vi "Server FGV.vi"(7 "Mode (Get All)":T2=enum."Get All", 8 "error in (no error)":errorcluster, 11 "Stock Name":string) -> (0 "error out":errorcluster, 2 "purchase price":dbl, 3 "Full Features MCP Server Data":T1)   [LabVIEW 2025, in "Full Featured MCP Server.lvlib"]
doc: "This FGV contains the data for the stock market server. It makes sure no race-conditions happen when accessing the data in the main.vi and the mcp tools simultaneously."
uses:
  Server FGV Modes.ctl
  Server Data.ctl
  <vilib>/Utility/error.llb/Error Cluster From Error Code.vi
  <vilib>/ErrorRing/Error Ring.xnode
  Full Featured MCP Server.lvlib
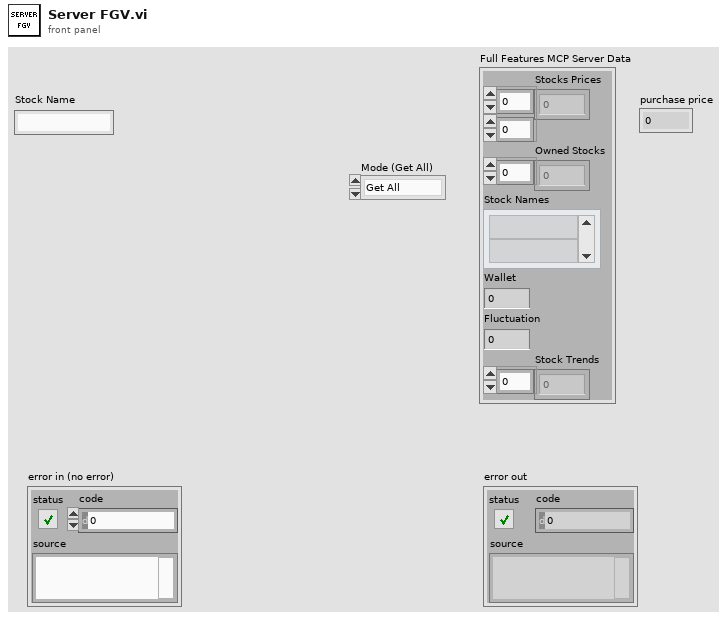
[diagram p1: front panel]
types:
  T1 = typedef "Full Featured MCP Server.lvlib/Server Data.ctl" = cluster{"Stocks Prices":dbl[][], "Owned Stocks":i32[], "Stock Names":string[], "Wallet":dbl, "Fluctuation":dbl, "Stock Trends":dbl[]}
  T2 = typedef "Full Featured MCP Server.lvlib/Server FGV Modes.ctl" = enum16{"Update Stocks", "Buy Stock", "Get All", "Init"}
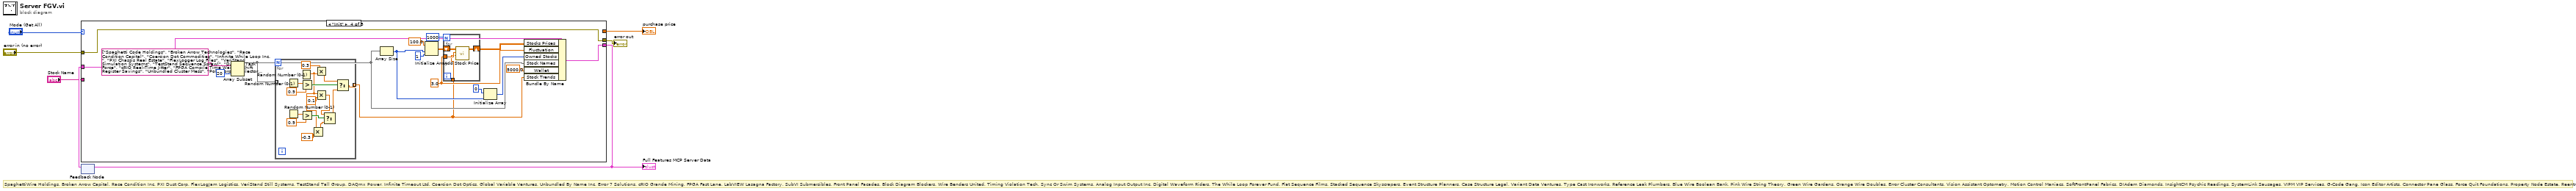
[diagram p0: block diagram]
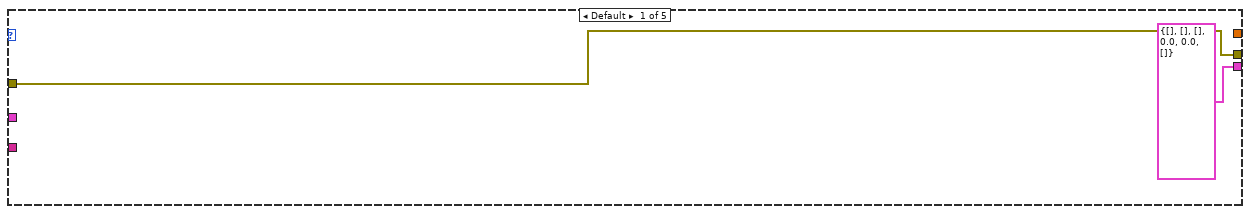
[diagram p2: hidden frame]
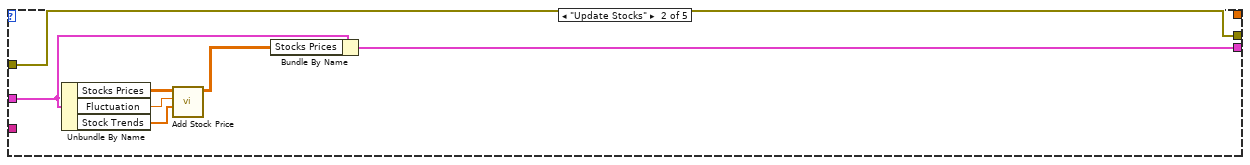
[diagram p3: hidden frame]
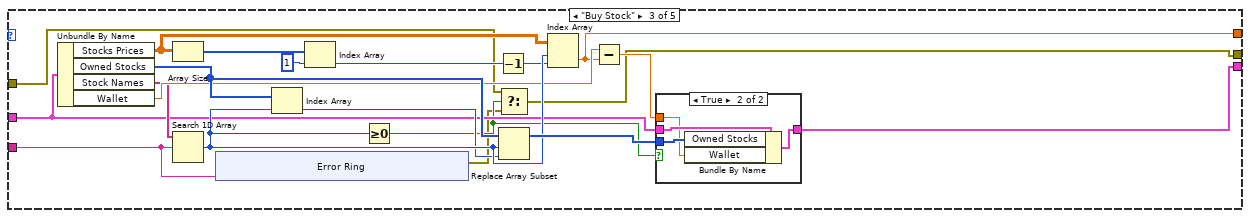
[diagram p4: hidden frame]
diagram:
  # "SpaghettiWire Holdings, Broken Arrow Capital, Race Condition Inc, PXI Dust Corp, FlexLogJam Logistics, VeriStand Still Systems, TestStand Tall Group, DAQmx Power, Infinite Timeout Ltd, Coercion Dot Optics, Global Variable Ventures, Unbundled By Name Inc, Error 7 Solutions, cRIO Grande Mining, FPGA Fast Lane, LabVIEW Lasagna Factory, SubVI Submersibles, Front Panel Facades, Block Diagram Blockers, Wire Benders United, Timing Violation Tech, Sync Or Swim Systems, Analog Input Output Inc, Digital Waveform Riders, The While Loop Forever Fund, Flat Sequence Films, Stacked Sequence Skyscrapers, Event Structure Planners, Case Structure Legal, Variant Data Ventures, Type Cast Ironworks, Reference Leak Plumbers, Blue Wire Boolean Bank, Pink Wire String Theory, Green Wire Gardens, Orange Wire Doubles, Error Cluster Consultants, Vision Assistant Optometry, Motion Control Maniacs, SoftFrontPanel Fabrics, DIAdem Diamonds, InsightCM Psychic Readings, SystemLink Sausages, VIPM VIP Services, G-Code Gang, Icon Editor Artists, Connector Pane Glass, Force Quit Foundations, Property Node Estate, Reentrant Execution Groups"
  n1 = feedback #1() -> (w6:T1)  [unwired: 1 in]
  n2 = case shown="\"Init\"" "Mode (Get All)" {
    tunnel: [T1 {"Stocks Prices"=[], "Owned Stocks"=[], "Stock Names"=[], "Wallet"=0.0, "Fluctuation"=0.0, "Stock Trends"=[]} ("Full Features MCP Server Data") w16 w24 w63 w86] -> w5
    tunnel: w6 -> [_ w15 w23 w65 w86]
    tunnel: "Stock Name" -> [_ _ w17 _ _]
    tunnel: [_ _ w22 _ _] -> w3
    tunnel: "error in (no error)" -> [w8 w11 w21 w64 w85]
    tunnel: [w8 w11 w20 w64 w85] -> w1
    frame Default {
    }
    frame "Update Stocks" {
      n3 = Unbundle By Name(w15) -> ("Stocks Prices"=w14:dbl[][], "Fluctuation"=w13:dbl, "Stock Trends"=w10:dbl[])
      n4 = call "Add Stock Price.vi"("Trends"=w10, "Fluctuation"=w13, "Stocks Prices"=w14) -> ("Stock Prices out"=w12:dbl[][])  [unwired: 8 in]
      n5 = Bundle By Name(cluster=w15, "Stocks Prices"=w12) -> (w16:T1)
    }
    frame "Buy Stock" {
      n6 = Unbundle By Name(w23) -> ("Stocks Prices"=w26:dbl[][], "Owned Stocks"=w32:i32[], "Stock Names"=w25:string[], "Wallet"=w31:dbl)
      n7 = Array Size(array=w26) -> (size(s)=w27:i32[])
      n8 = Search 1D Array(1D array=w25, element=w17) -> (index of element=w34:i32)  [unwired: 1 in]
      n9 = xnode "Error Ring"("parameter 0"=w17) -> ("error out"=w18:errorcluster)
      n10 = Index Array(array=w32, index=w34) -> (element=w33:i32)
      n11 = Index Array(array=w27, index=1) -> (element=w29:i32)
      n12 = Greater Or Equal To 0?(x=w34) -> (x >= 0?=w19:bool)
      n13 = Decrement(x=w29) -> (x-1=w28:i32)
      n14 = Select(t=w21, s=w19, f=w18) -> (s? t:f=w20:errorcluster)
      n15 = Replace Array Subset(array=w32, new element=w33, index=w34) -> (w35:i32[])
      n16 = Index Array(array=w26, index (row)=w34, index (col)=w28) -> (element=w22:dbl)
      n17 = Subtract(x=w31, y=w22) -> (x-y=w36:dbl)
      n18 = case shown="True" w19 {
        tunnel: w23 -> [w44 w48]
        tunnel: w35 -> [_ w47]
        tunnel: w36 -> [_ w46]
        tunnel: [w44 w45] -> w24
        frame False {
        }
        frame True {
          n19 = Bundle By Name(cluster=w48, "Owned Stocks"=w47, "Wallet"=w46) -> (w45:T1)
        }
      }
    }
    frame "Init" {
      w60 = 3.0 ("Fluctuation")
      n20 = Array Subset(array=string[] ["Spaghetti Code Holdings", "Broken Arrow Technologies", "Race Condition Capital", "Coercion Dot Commodities", "Infinite While Loop Inc.", "PXI Chassis Real Estate", "FlexLogger Log Files", "VeriStand Simulation Systems", "TestStand Sequence Sprawl", "DAQmx Task Force", "cRIO Real-Time Jitter", "FPGA Compile Time Waits", "Shift Register Savings", "Unbundled Cluster Mess", "Polymorphic Selector Group", "SubVI Reentrancy Labs", "Global Variable Chaos", "Local Variable Abuse Co.", "Flat Sequence Films", "Stacked Sequence Mysteries", "Measurement & Automation X", "GPIB Cable Anchors", "VISA Resource Unknowns", "Serial Port Baud Rates", "Trigger Line Triggers", "Waveform Graph Aesthetics", "Chart History Buffers", "Dynamic Data Type Unknowns", "Variant To Data Casts", "Reference Leak Inc.", "Garbage Collection Denial", "Front Panel Cosmetics", "Block Diagram Sprawl", "Icon Editor Pixels", "Connector Pane Patterns", "Strict Type Def Corp.", "Auto-Indexing Tunnels", "Case Structure Defaults", "Event Structure Timeouts", "Producer Consumer Queues", "State Machine Logic", "Notifier Notifications", "Semaphore Lockouts", "Rendezvous Timing", "First Call Primitives", "Property Node Performance", "Invoke Node Methods", "Missing Driver Logistics", "License Manager Servers", "Error 42 Enterprises"] ("Array 3"), length=20) -> (w50:string[])  [unwired: 1 in]
      n21 = for {
        tunnel: w50 -> [_] mode=indexing
        tunnel: [w66] -> w49 mode=indexing
        n22 = Random Number (0-1)() -> (number: 0 to 1=w80:dbl)
        n23 = Random Number (0-1)() -> (number: 0 to 1=w73:dbl)
        n24 = Random Number (0-1)() -> (number: 0 to 1=w67:dbl)
        n25 = Greater?(x=w80, y=0.9) -> (0:w78:bool)
        n26 = Greater?(x=w73, y=0.9) -> (0:w72:bool)
        n27 = Multiply(x=w67, y=-0.3) -> (x*y=w68:dbl)
        n28 = Multiply(x=0.3, y=w67) -> (x*y=w76:dbl)
        n29 = Multiply(x=w67, y=0.1) -> (x*y=w70:dbl)
        n30 = Select(t=w70, s=w72, f=w68) -> (s? t:f=w71:dbl)
        n31 = Select(t=w76, s=w78, f=w71) -> (s? t:f=w66:dbl)
      }
      n32 = Array Size(array=w50) -> (size(s)=w55:i32)
      n33 = Initialize Array(100.0 ("element"), w55, 1 ("dimension size")) -> (w57:dbl[][])
      n34 = for {
        N: 1000 -> [_]
        tunnel: w60 -> [w83]
        shift-right: [w84] -> w61
        shift-left: w57 -> [w82]
        tunnel: w49 -> [w81]
        n35 = call "Add Stock Price.vi"("Trends"=w81, "Fluctuation"=w83, "Stocks Prices"=w82) -> ("Stock Prices out"=w84:dbl[][])  [unwired: 8 in]
      }
      n36 = Initialize Array(0 ("element"), w55) -> (w54:i32[])
      n37 = Bundle By Name(cluster=w65, "Stocks Prices"=w61, "Fluctuation"=w60, "Owned Stocks"=w54, "Stock Names"=w50, "Wallet"=5000.0, "Stock Trends"=w49) -> (w63:T1)
    }
    frame "Get All" {
    }
  }
  "Full Features MCP Server Data" <- w5
  "error out" <- w1
  "purchase price" <- w3
  n38 = feedback-in #1(w5) -> ()
